vi "Get Desired Size.vi"(8 "error in (no error)":errorcluster, 11 "PlatformArrayPanel in":refnum<class "PlatformArrayPanel.lvclass">) -> (0 "error out":errorcluster, 2 "Desired Size":T1, 3 "PlatformArrayPanel out":refnum<class "PlatformArrayPanel.lvclass">)   [LabVIEW 2020, in "PicoG-App.lvlib" / "PlatformArrayPanel.lvclass"]
uses:
  PlatformArrayPanel.lvclass
  <vilib>/IlluminatedG/IG OOPanel/OOPanel/ArrayPanel/Desired Size.ctl
  <vilib>/IlluminatedG/IG OOPanel/OOPanel/OOPanel.lvlib
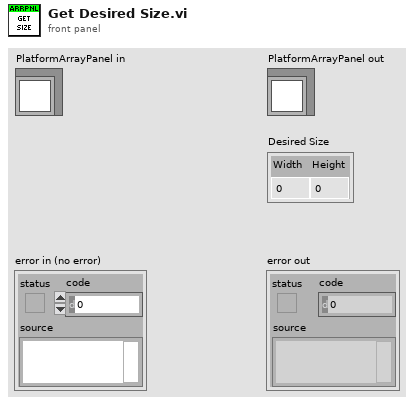
[diagram p1: front panel]
types:
  T1 = typedef "OOPanel.lvlib/Desired Size.ctl" = cluster{"Width":u32, "Height":u32}
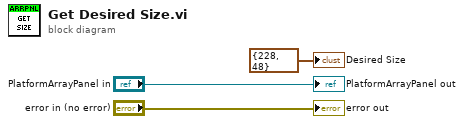
[diagram p0: block diagram]
diagram:
  "error out" <- "error in (no error)"
  "PlatformArrayPanel out" <- "PlatformArrayPanel in"
  "Desired Size" <- T1 {"Width"=228, "Height"=48} ("Desired Size")
